vi "Renew QDFunctions Library.vi"(8 "error in (no error)":errorcluster, 10 "QDFunction Path":path, 11 "ScriptSetting in":refnum<class "ScriptSetting.lvclass">) -> (0 "error out":errorcluster, 3 "ScriptSetting out":refnum<class "ScriptSetting.lvclass">)   [LabVIEW 2015, in "ScriptSetting.lvclass"]
uses:
  ScriptSetting.lvclass
  ScriptSetting.lvclass/ScriptSetting.ctl
  _Database/Implements/ScriptDatabase.lvclass/ScriptDatabase.ctl
  QDSearchList/QDDialogList.lvclass/QDDialogList.ctl
  QDSearchList/QDDialogList.lvclass
  _Database/Ancestor/DatabaseAPI.lvclass
  _Database/Implements/ScriptDatabase.lvclass
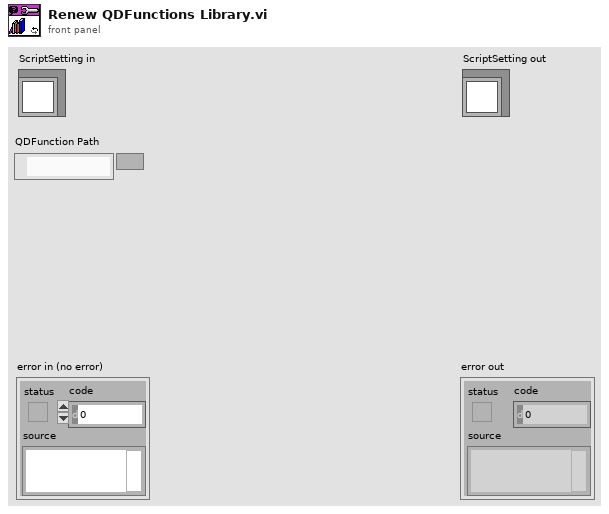
[diagram p1: front panel]
types:
  T1 = cluster{"[0]":string, "[1]":string, "[2]":string}
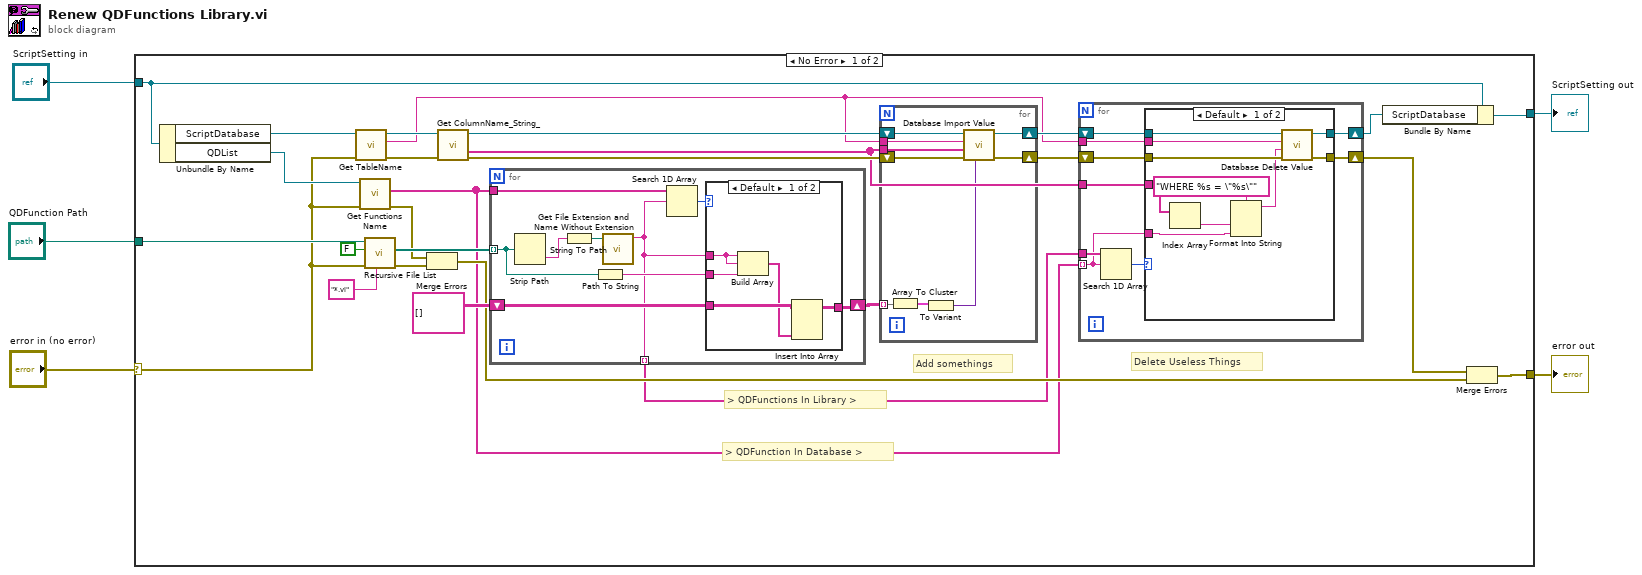
[diagram p0: block diagram]
diagram:
  n1 = case shown="No Error" "error in (no error)" {
    selector: "error in (no error)" -> [w23 w79]
    tunnel: [w15 w79] -> w4
    tunnel: [w17 w78] -> w2
    tunnel: "ScriptSetting in" -> [w20 w78]
    tunnel: "QDFunction Path" -> [w32 _]
    frame No Error {
      # "> QDFunction In Database >"
      # "> QDFunctions In Library >"
      # "Delete Useless Things"
      # "Add somethings"
      n2 = Unbundle By Name(w20) -> ("ScriptDatabase"=w24:refnum<class "ScriptDatabase.lvclass">, "QDList"=w28:refnum<class "QDDialogList.lvclass">)
      n3 = call "Get TableName.vi"("error in (no error)"=w23, "ScriptDatabase in"=w24) -> ("error out"=w21:errorcluster, "TableName"=w10:string, "ScriptDatabase out"=w22:refnum<class "ScriptDatabase.lvclass">)  [unwired: 7 in]
      n4 = call "Get Functions Name.vi"("error in (no error)"=w23, "QDDialogList in"=w28) -> ("error out"=w26:errorcluster, "Functions Name"=w11:string[])  [unwired: 7 in, 1 out]
      n5 = call <vilib>:"Recursive File List.vi"("pattern"="*.vi", "error in (no error)"=w23, "Treat LLBs as Folders?"=FALSE, "Folder Path"=w32) -> ("error out"=w27:errorcluster, "All Files in Dir"=w29:path[])  [unwired: 3 in, 3 out]
      n6 = Merge Errors(w26, w27) -> (w16:errorcluster)
      n7 = call "Get ColumnName_String_.vi"("error in (no error)"=w21, "ScriptDatabase in"=w22) -> ("error out"=w19:errorcluster, "ColumnName<String>"=w9:string[], "ScriptDatabase out"=w18:refnum<class "ScriptDatabase.lvclass">)  [unwired: 7 in]
      n8 = for {
        tunnel: w29 -> [w70] mode=indexing
        tunnel: w11 -> [w71]
        shift-right: [w67] -> w14
        shift-left: string[][] [] -> [w68]
        tunnel: [w63] -> w6 mode=indexing
        n9 = Strip Path(path=w70) -> (name=w65:string)  [unwired: 1 out]
        n10 = String To Path(string=w65) -> (path=w64:path)
        n11 = Path To String(path=w70) -> (string=w69:string)
        n12 = call <userlib>:"Get File Extension and Name Without Extension.vi"("file"=w64) -> ("filename without extension"=w63:string)  [unwired: 9 in, 1 out]
        n13 = Search 1D Array(1D array=w71, element=w63) -> (index of element=w66:i32)  [unwired: 1 in]
        n14 = case shown="Default" w66 {
          tunnel: w63 -> [w76 _]
          tunnel: w69 -> [w75 _]
          tunnel: w68 -> [w74 w77]
          tunnel: [w72 w77] -> w67
          frame Default {
            n15 = Build Array(w76, w76, w75) -> (w73:string[])
            n16 = Insert Into Array(array=w74, new element=w73) -> (w72:string[][])  [unwired: 2 in]
          }
          frame 0.. {
          }
        }
      }
      n17 = for {
        tunnel: w10 -> [w62]
        tunnel: w9 -> [w61]
        shift-right: [w57] -> w12
        shift-left: w19 -> [w60]
        shift-right: [w58] -> w13
        shift-left: w18 -> [w59]
        tunnel: w14 -> [w54] mode=indexing
        n18 = Array To Cluster(array=w54) -> (cluster=w56:T1)
        n19 = To Variant(anything=w56) -> (Variant=w55:variant)
        n20 = call "Database Import Value.vi"("data"=w55, "error in (no error)"=w60, "columns"=w61, "table"=w62, "object in"=w59) -> ("error out"=w57:errorcluster, "object out"=w58:refnum<class "ScriptDatabase.lvclass">)  [unwired: 5 in]
      }
      n21 = for {
        tunnel: w11 -> [w39] mode=indexing
        tunnel: w6 -> [w41]
        shift-right: [w36] -> w7
        shift-left: w13 -> [w37]
        tunnel: w10 -> [w34]
        tunnel: w9 -> [w35]
        shift-right: [w33] -> w8
        shift-left: w12 -> [w38]
        n22 = Search 1D Array(1D array=w41, element=w39) -> (index of element=w40:i32)  [unwired: 1 in]
        n23 = case shown="Default" w40 {
          tunnel: w39 -> [w44 _]
          tunnel: w38 -> [w50 w52]
          tunnel: w37 -> [w51 w53]
          tunnel: [w49 w53] -> w36
          tunnel: w35 -> [w46 _]
          tunnel: w34 -> [w47 _]
          tunnel: [w42 w52] -> w33
          frame Default {
            n24 = Index Array(array=w46) -> (element=w45:string)  [unwired: 1 in]
            n25 = Format Into String(format string="WHERE %s = \"%s\"", w45, w44) -> (resulting string=w43:string)  [unwired: 2 in, 1 out]
            n26 = call "Database Delete Value.vi"("error in (no error)"=w50, "condition"=w43, "table"=w47, "object in"=w51) -> ("error out"=w42:errorcluster, "object out"=w49:refnum<class "ScriptDatabase.lvclass">)  [unwired: 6 in]
          }
          frame 0.. {
          }
        }
      }
      n27 = Bundle By Name(cluster=w20, "ScriptDatabase"=w7) -> (w17:refnum<class "ScriptSetting.lvclass">)
      n28 = Merge Errors(w8, w16) -> (w15:errorcluster)
    }
    frame Error {
    }
  }
  "error out" <- w4
  "ScriptSetting out" <- w2
